vi "Get or Add Font.vi"(8 "error in":errorcluster, 10 "Fonts":T1={"Bold"=enum."default", "Italic"=enum."default", "Underline"=enum."default", "Color"=0, "Size"=-1.0, "Name"=""}, 11 "SpreadsheetDoc in":refnum<k24>) -> (0 "error out":errorcluster, 1 "Font Id":i32, 2 "Font":refnum<k24>, 3 "SpreadsheetDoc out":refnum<k24>)   [LabVIEW 2021, in "Open Xml.lvlib"]
uses:
  Open Xml.lvlib
  D:/git/Open-Xml-LabVIEW/dll/DocumentFormat.OpenXml.dll
  dll/DocumentFormat.OpenXml.dll
  D:/git/Open-Xml-LabVIEW/dll/DocumentFormat.OpenXml.Framework.dll
  dll/DocumentFormat.OpenXml.Framework.dll
  190fa438-8aef-4082-9b70-6491aa84baf9.vi
  Font.ctl
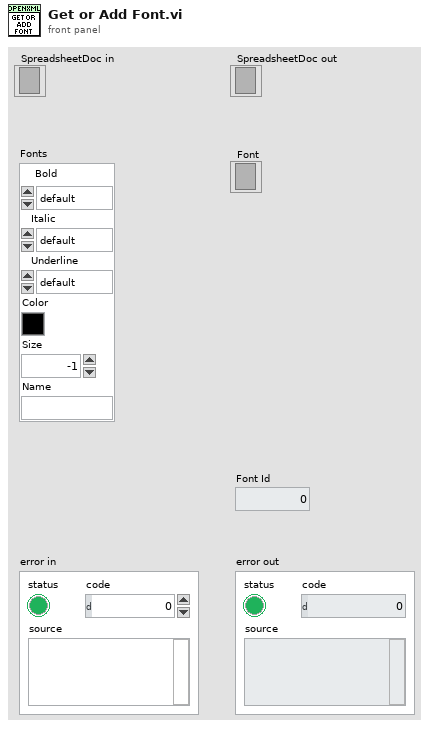
[diagram p1: front panel]
types:
  T1 = typedef "Open Xml.lvlib/Font.ctl" = cluster{"Bold":enum16{"bold", "regular", "default"}, "Italic":enum16{"italic", "regular", "default"}, "Underline":enum16{"single", "double", "singleAccounting", "doubleAccounting", "none", "default"}, "Color":u32, "Size":dbl, "Name":string}
  T2 = enum16{"Bold", "Italic", "Underline", "Color", "Size", "Name"}
  T3 = enum16{"Bold", "Italic", "Underline", "Color", "Size", "Name"}[]
  T4 = enum16{"single", "double", "singleAccounting", "doubleAccounting", "none", "default"}
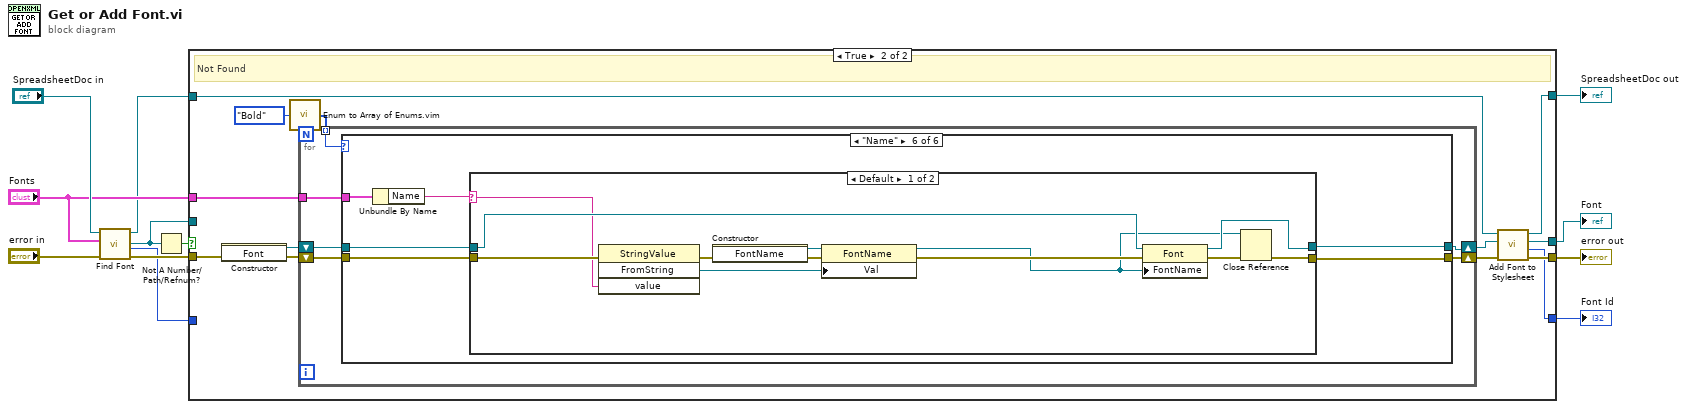
[diagram p0: block diagram]
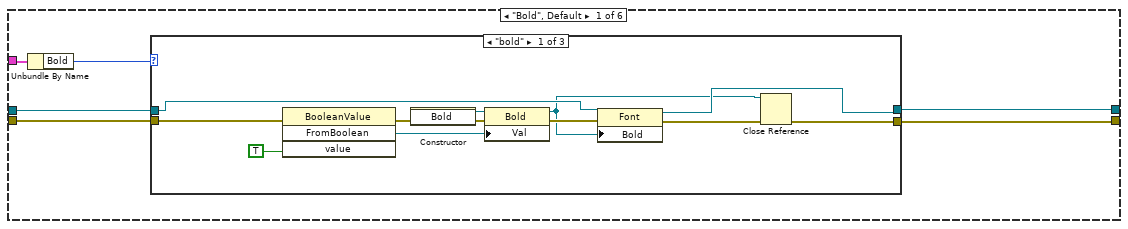
[diagram p3: hidden frame]
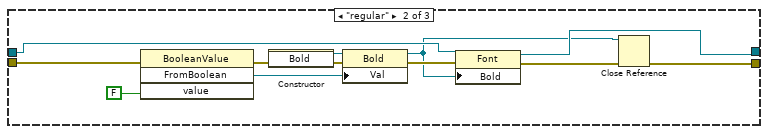
[diagram p4: hidden frame]
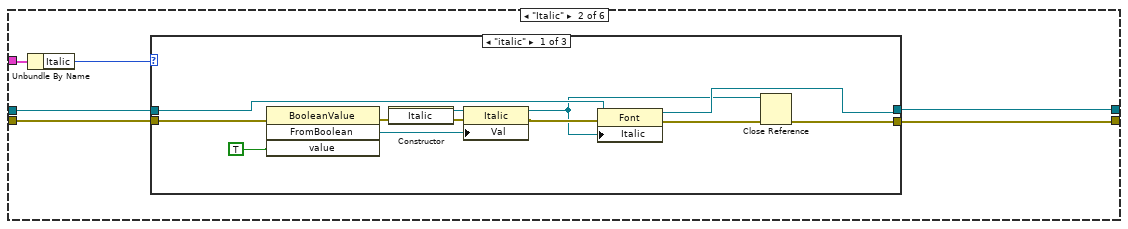
[diagram p6: hidden frame]
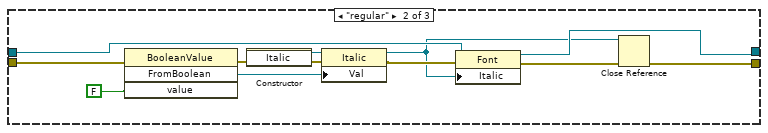
[diagram p7: hidden frame]
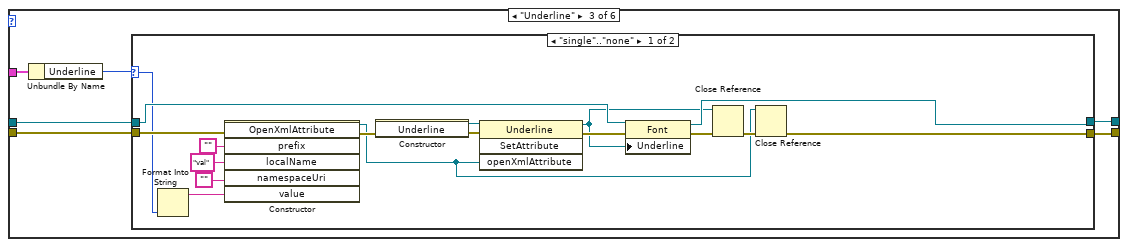
[diagram p9: hidden frame]
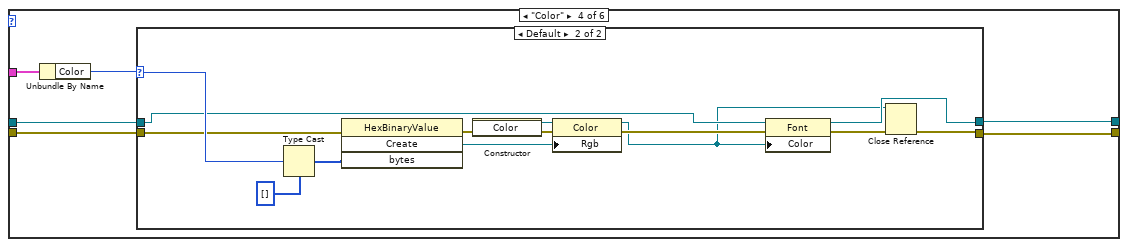
[diagram p11: hidden frame]
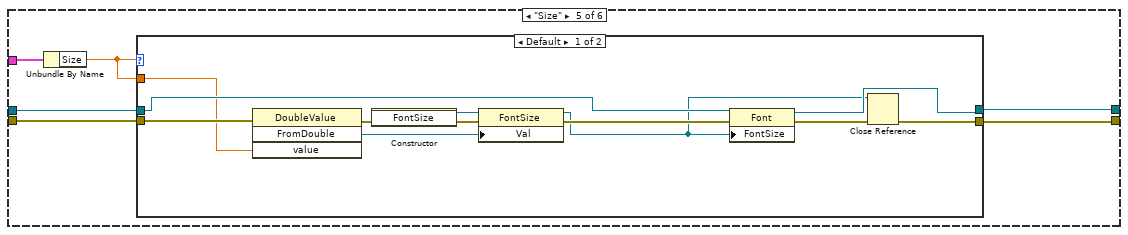
[diagram p13: hidden frame]
diagram:
  n1 = call "Find Font.vi"("error in"="error in", "Font"="Fonts", "SpreadsheetDoc in"="SpreadsheetDoc in") -> ("error out"=w10:errorcluster, "FontId"=w5:i32, "Font"=w8:refnum<k24>, "SpreadsheetDoc out"=w3:refnum<k24>)  [unwired: 5 in]
  n2 = Not A Number/Path/Refnum?(number/path/refnum=w8) -> (NaN/Path/Refnum?=w9:bool)
  n3 = case shown="True" w9 {
    tunnel: w10 -> [w16 w17]
    tunnel: w8 -> [w14 _]
    tunnel: "Fonts" -> [_ w29]
    tunnel: [w16 w23] -> w7
    tunnel: w5 -> [w15 _]
    tunnel: [w15 w20] -> w4
    tunnel: w3 -> [w13 w18]
    tunnel: [w13 w19] -> w2
    tunnel: [w14 w21] -> w1
    frame False {
      # "Found"
    }
    frame True {
      # "Not Found"
      n4 = constructor class="Font"(error in=w17) -> (reference out=w24:refnum<k24>, error out=w25:errorcluster)  [unwired: 2 in, 1 out]
      n5 = call "Enum to Array of Enums.vim"("enum"=T2."Bold") -> ("array of enums"=w26:T3)
      n6 = for {
        tunnel: w29 -> [w35]
        shift-right: [w33] -> w28
        shift-left: w25 -> [w34]
        tunnel: w26 -> [w32] mode=indexing
        shift-right: [w30] -> w22
        shift-left: w24 -> [w31]
        n7 = case shown="\"Name\"" w32 {
          tunnel: w35 -> [w40 w72 w104 w129 w151 w171]
          tunnel: w34 -> [w41 w73 w105 w130 w152 w172]
          tunnel: [w37 w69 w101 w126 w149 w168] -> w33
          tunnel: w31 -> [w38 w70 w102 w127 w150 w169]
          tunnel: [w36 w68 w100 w125 w148 w167] -> w30
          frame "Bold", Default {
            n8 = Unbundle By Name(w40) -> ("Bold"=w39:enum16{"bold", "regular", "default"})
            n9 = case shown="\"bold\"" w39 {
              tunnel: w41 -> [w49 w61 w67]
              tunnel: w38 -> [w47 w59 w66]
              tunnel: [w43 w55 w67] -> w37
              tunnel: [w44 w56 w66] -> w36
              frame "bold" {
                n10 = invoke class="BooleanValue" method="FromBoolean"(error in=w49, "value"=TRUE) -> (error out=w51:errorcluster, "FromBoolean"=w50:refnum<k24>)  [unwired: 2 in, 2 out]
                n11 = constructor class="Bold"(error in=w51) -> (reference out=w53:refnum<k24>, error out=w52:errorcluster)  [unwired: 2 in, 1 out]
                n12 = property class="Bold"(reference=w53, error in=w52, "Val"=w50) -> (reference out=w42:refnum<k24>, error out=w46:errorcluster)
                n13 = property class="Font"(reference=w47, error in=w46, "Bold"=w42) -> (reference out=w44:refnum<k24>, error out=w45:errorcluster)
                n14 = Close Reference(reference=w42, error in (no error)=w45) -> (error out=w43:errorcluster)
              }
              frame "regular" {
                n15 = invoke class="BooleanValue" method="FromBoolean"(error in=w61, "value"=FALSE) -> (error out=w63:errorcluster, "FromBoolean"=w62:refnum<k24>)  [unwired: 2 in, 2 out]
                n16 = constructor class="Bold"(error in=w63) -> (reference out=w65:refnum<k24>, error out=w64:errorcluster)  [unwired: 2 in, 1 out]
                n17 = property class="Bold"(reference=w65, error in=w64, "Val"=w62) -> (reference out=w54:refnum<k24>, error out=w58:errorcluster)
                n18 = property class="Font"(reference=w59, error in=w58, "Bold"=w54) -> (reference out=w56:refnum<k24>, error out=w57:errorcluster)
                n19 = Close Reference(reference=w54, error in (no error)=w57) -> (error out=w55:errorcluster)
              }
              frame "default", Default {
              }
            }
          }
          frame "Italic" {
            n20 = Unbundle By Name(w72) -> ("Italic"=w71:enum16{"italic", "regular", "default"})
            n21 = case shown="\"italic\"" w71 {
              tunnel: w73 -> [w78 w90 w99]
              tunnel: w70 -> [w77 w89 w98]
              tunnel: [w83 w95 w99] -> w69
              tunnel: [w84 w96 w98] -> w68
              frame "italic" {
                n22 = invoke class="BooleanValue" method="FromBoolean"(error in=w78, "value"=TRUE) -> (error out=w82:errorcluster, "FromBoolean"=w79:refnum<k24>)  [unwired: 2 in, 2 out]
                n23 = constructor class="Italic"(error in=w82) -> (reference out=w80:refnum<k24>, error out=w81:errorcluster)  [unwired: 2 in, 1 out]
                n24 = property class="Italic"(reference=w80, error in=w81, "Val"=w79) -> (reference out=w75:refnum<k24>, error out=w76:errorcluster)
                n25 = property class="Font"(reference=w77, error in=w76, "Italic"=w75) -> (reference out=w84:refnum<k24>, error out=w85:errorcluster)
                n26 = Close Reference(reference=w75, error in (no error)=w85) -> (error out=w83:errorcluster)
              }
              frame "regular" {
                n27 = invoke class="BooleanValue" method="FromBoolean"(error in=w90, "value"=FALSE) -> (error out=w94:errorcluster, "FromBoolean"=w91:refnum<k24>)  [unwired: 2 in, 2 out]
                n28 = constructor class="Italic"(error in=w94) -> (reference out=w92:refnum<k24>, error out=w93:errorcluster)  [unwired: 2 in, 1 out]
                n29 = property class="Italic"(reference=w92, error in=w93, "Val"=w91) -> (reference out=w87:refnum<k24>, error out=w88:errorcluster)
                n30 = property class="Font"(reference=w89, error in=w88, "Italic"=w87) -> (reference out=w96:refnum<k24>, error out=w97:errorcluster)
                n31 = Close Reference(reference=w87, error in (no error)=w97) -> (error out=w95:errorcluster)
              }
              frame "default", Default {
              }
            }
          }
          frame "Underline" {
            n32 = Unbundle By Name(w104) -> ("Underline"=w103:T4)
            n33 = case shown="\"single\"..\"none\"" w103 {
              selector: w103 -> [w112 _]
              tunnel: w105 -> [w114 w124]
              tunnel: w102 -> [w118 w123]
              tunnel: [w107 w124] -> w101
              tunnel: [w121 w123] -> w100
              frame "single".."none" {
                n34 = Format Into String(w112) -> (resulting string=w110:string)  [unwired: 3 in, 1 out]
                n35 = constructor class="OpenXmlAttribute"(error in=w114, "prefix"="", "localName"="val" ("prefix"), "namespaceUri"="", "value"=w110) -> (reference out=w106:refnum<k24>, error out=w113:errorcluster)  [unwired: 2 in, 5 out]
                n36 = constructor class="Underline"(error in=w113) -> (reference out=w119:refnum<k24>, error out=w120:errorcluster)  [unwired: 2 in, 1 out]
                n37 = invoke class="Underline" method="SetAttribute"(reference=w119, error in=w120, "openXmlAttribute"=w106) -> (reference out=w115:refnum<k24>, error out=w117:errorcluster)  [unwired: 1 in, 2 out]
                n38 = property class="Font"(reference=w118, error in=w117, "Underline"=w115) -> (reference out=w121:refnum<k24>, error out=w122:errorcluster)
                n39 = Close Reference(reference=w115, error in (no error)=w122) -> (error out=w116:errorcluster)
                n40 = Close Reference(reference=w106, error in (no error)=w116) -> (error out=w107:errorcluster)
              }
              frame "default", Default {
              }
            }
          }
          frame "Color" {
            n41 = Unbundle By Name(w129) -> ("Color"=w128:u32)
            n42 = case shown="Default" w128 {
              selector: w128 -> [_ w140]
              tunnel: w130 -> [w132 w139]
              tunnel: w127 -> [w131 w136]
              tunnel: [w132 w134] -> w126
              tunnel: [w131 w135] -> w125
              frame 16777216 {
                # "Transparent is chosen to mean default"
              }
              frame Default {
                n43 = Type Cast(type=u8[] [], x=w140) -> (*(type *) &x=w142:u8[])
                n44 = invoke class="HexBinaryValue" method="Create"(error in=w139, "bytes"=w142) -> (error out=w141:errorcluster, "Create"=w144:refnum<k24>)  [unwired: 2 in, 2 out]
                n45 = constructor class="Color"(error in=w141) -> (reference out=w146:refnum<k24>, error out=w145:errorcluster)  [unwired: 2 in, 1 out]
                n46 = property class="Color"(reference=w146, error in=w145, "Rgb"=w144) -> (reference out=w133:refnum<k24>, error out=w138:errorcluster)
                n47 = property class="Font"(reference=w136, error in=w138, "Color"=w133) -> (reference out=w135:refnum<k24>, error out=w137:errorcluster)
                n48 = Close Reference(reference=w133, error in (no error)=w137) -> (error out=w134:errorcluster)
              }
            }
          }
          frame "Size" {
            n49 = Unbundle By Name(w151) -> ("Size"=w147:dbl)
            n50 = case shown="Default" w147 {
              tunnel: w152 -> [w158 w165]
              tunnel: w150 -> [w157 w166]
              tunnel: [w154 w165] -> w149
              tunnel: [w163 w166] -> w148
              tunnel: w147 -> [w155 _]
              frame Default {
                n51 = invoke class="DoubleValue" method="FromDouble"(error in=w158, "value"=w155) -> (error out=w160:errorcluster, "FromDouble"=w161:refnum<k24>)  [unwired: 2 in, 2 out]
                n52 = constructor class="FontSize"(error in=w160) -> (reference out=w162:refnum<k24>, error out=w159:errorcluster)  [unwired: 2 in, 1 out]
                n53 = property class="FontSize"(reference=w162, error in=w159, "Val"=w161) -> (reference out=w153:refnum<k24>, error out=w156:errorcluster)
                n54 = property class="Font"(reference=w157, error in=w156, "FontSize"=w153) -> (reference out=w163:refnum<k24>, error out=w164:errorcluster)
                n55 = Close Reference(reference=w153, error in (no error)=w164) -> (error out=w154:errorcluster)
              }
              frame ..0 {
              }
            }
          }
          frame "Name" {
            n56 = Unbundle By Name(w171) -> ("Name"=w170:string)
            n57 = case shown="Default" w170 {
              selector: w170 -> [w175 _]
              tunnel: w172 -> [w177 w186]
              tunnel: w169 -> [w182 w185]
              tunnel: [w174 w186] -> w168
              tunnel: [w183 w185] -> w167
              frame Default {
                n58 = invoke class="StringValue" method="FromString"(error in=w177, "value"=w175) -> (error out=w178:errorcluster, "FromString"=w180:refnum<k24>)  [unwired: 2 in, 2 out]
                n59 = constructor class="FontName"(error in=w178) -> (reference out=w181:refnum<k24>, error out=w179:errorcluster)  [unwired: 2 in, 1 out]
                n60 = property class="FontName"(reference=w181, error in=w179, "Val"=w180) -> (reference out=w173:refnum<k24>, error out=w176:errorcluster)
                n61 = property class="Font"(reference=w182, error in=w176, "FontName"=w173) -> (reference out=w183:refnum<k24>, error out=w184:errorcluster)
                n62 = Close Reference(reference=w173, error in (no error)=w184) -> (error out=w174:errorcluster)
              }
              frame "" {
              }
            }
          }
        }
      }
      n63 = call "Add Font to Stylesheet.vi"("error in"=w28, "Font in"=w22, "SpreadsheetDoc in"=w18) -> ("error out"=w23:errorcluster, "Index"=w20:i32, "Font out"=w21:refnum<k24>, "SpreadsheetDoc out"=w19:refnum<k24>)  [unwired: 5 in]
    }
  }
  "SpreadsheetDoc out" <- w2
  "error out" <- w7
  "Font" <- w1
  "Font Id" <- w4
